vi "Tank Fills Gradually.vi"() -> ()   [LabVIEW 2016]
panel:
  out "Tank":dbl(slide) scale=0.0..100.0
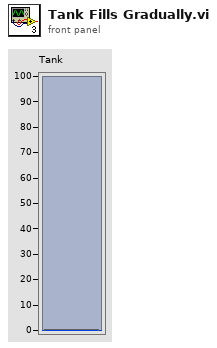
[diagram p1: front panel]
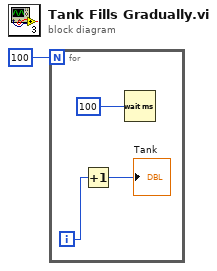
[diagram p0: block diagram]
diagram:
  n1 = for {
    N: 100 ("Numeric") -> [_]
    i -> [w4]
    n2 = Increment(x=w4) -> (x+1=→"Tank":i32)
    n3 = Wait (ms)(milliseconds to wait=100) -> ()  [unwired: 1 out]
  }
